vi "FlatToRichni_bus_monitor_api_ConnectSettings.vi"(5 "OutputClusterType":T1, 11 "InputCluster":T5) -> (3 "OutputCluster":T1)   [LabVIEW 2025, in "bus_monitor_client.lvlib"]
uses:
  ni_bus_monitor_api_ConnectSettings_Flat.ctl
  ni_bus_monitor_api_CanMode.ctl
  ni_bus_monitor_api_Termination.ctl
  ni_bus_monitor_api_FdIsoMode.ctl
  ni_bus_monitor_api_ConnectSettings.ctl
  bus_monitor_client.lvlib
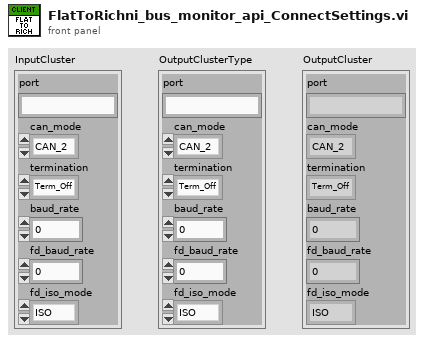
[diagram p1: front panel]
types:
  T1 = typedef "bus_monitor_client.lvlib/ni_bus_monitor_api_ConnectSettings.ctl" = cluster{"port":string, "can_mode":T2, "termination":T3, "baud_rate":u64, "fd_baud_rate":u64, "fd_iso_mode":T4}
  T2 = typedef "bus_monitor_client.lvlib/ni_bus_monitor_api_CanMode.ctl" = enum32{"CAN_2", "CAN_FD", "CAN_FD_BRS"}
  T3 = typedef "bus_monitor_client.lvlib/ni_bus_monitor_api_Termination.ctl" = enum32{"Term_Off", "Term_On"}
  T4 = typedef "bus_monitor_client.lvlib/ni_bus_monitor_api_FdIsoMode.ctl" = enum32{"ISO", "Non_ISO", "ISO_Legacy"}
  T5 = typedef "bus_monitor_client.lvlib/ni_bus_monitor_api_ConnectSettings_Flat.ctl" = cluster{"port":string, "can_mode":T2, "termination":T3, "baud_rate":u64, "fd_baud_rate":u64, "fd_iso_mode":T4}
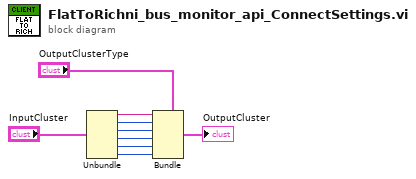
[diagram p0: block diagram]
diagram:
  n1 = Unbundle "Unbundle"("InputCluster") -> ("port"=w6:string, "can_mode"=w5:T2, "termination"=w4:T3, "baud_rate"=w3:u64, "fd_baud_rate"=w2:u64, "fd_iso_mode"=w1:T4)
  n2 = Bundle "Bundle"(cluster="OutputClusterType", "port"=w6, "can_mode"=w5, "termination"=w4, "baud_rate"=w3, "fd_baud_rate"=w2, "fd_iso_mode"=w1) -> (→"OutputCluster":T1)
